vi "Filename Generator.vi"(9 "Measurement Type":string, 10 "Sample Properties:":T1, 11 "Saved Folder:":path=path "C:/1DATA/2011") -> (3 "Filepath Out":path)   [LabVIEW 2012]
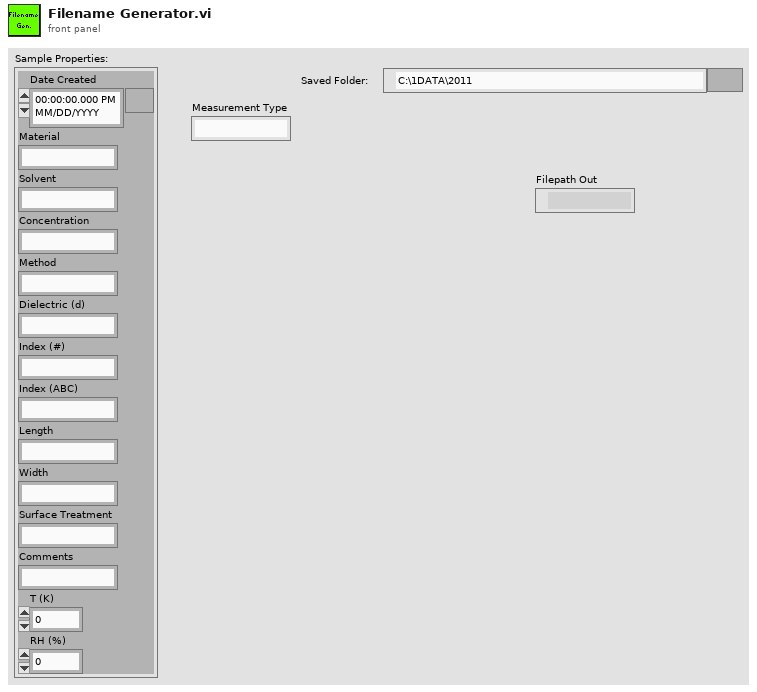
[diagram p1: front panel]
types:
  T1 = cluster{"Date Created":timestamp, "Material":string, "Solvent":string, "Concentration":string, "Method":string, "Dielectric (d)":string, "Index (#)":string, "Index (ABC)":string, "Length":string, "Width":string, "Surface Treatment":string, "Comments":string, "T (K)":dbl, "RH (%)":dbl}
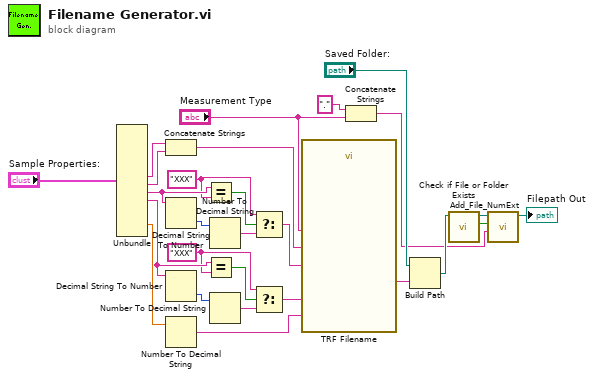
[diagram p0: block diagram]
diagram:
  w22 = "XXX"
  w19 = "XXX"
  n1 = Unbundle("Sample Properties:") -> ("Index (#)"=w14:string, "Index (ABC)"=w15:string, "Length"=w25:string, "Width"=w23:string, "T (K)"=w26:dbl)  [unwired: 9 out]
  n2 = Concatenate Strings(w14, w15) -> (w6:string)
  n3 = Decimal String To Number(string=w25) -> (number=w16:i32)  [unwired: 2 in, 1 out]
  n4 = Decimal String To Number(string=w23) -> (number=w17:i32)  [unwired: 2 in, 1 out]
  n5 = Number To Decimal String(number=w26) -> (decimal integer string=w2:string)  [unwired: 1 in]
  n6 = Equal?(x=w25, y=w19) -> (x = y?=w18:bool)
  n7 = Equal?(x=w23, y=w22) -> (x = y?=w21:bool)
  n8 = Number To Decimal String(number=w16) -> (decimal integer string=w20:string)  [unwired: 1 in]
  n9 = Number To Decimal String(number=w17) -> (decimal integer string=w24:string)  [unwired: 1 in]
  n10 = Select(t=w19, s=w18, f=w20) -> (s? t:f=w4:string)
  n11 = Select(t=w22, s=w21, f=w24) -> (s? t:f=w3:string)
  n12 = call "TRF Filename"("Width"=w3, "Type"="Measurement Type", "Index"=w6, "Length"=w4, "T"=w2) -> ("Result"=w13:string)  [unwired: 9 in, 1 out]
  n13 = Concatenate Strings("." ("string"), "Measurement Type") -> (w7:string)
  n14 = Build Path(base path="Saved Folder:", name or relative path=w13) -> (appended path=w11:path)
  n15 = call <vilib>:"Check if File or Folder Exists.vi"("path"=w11) -> ("file or folder exists?"=w10:bool, "dup path"=w9:path)  [unwired: 8 in, 1 out]
  n16 = call "Add_File_NumExt.vi"("Extension"=w7, "file or folder exists?"=w10, "Path In"=w9) -> ("Path Out"=→"Filepath Out":path)  [unwired: 8 in]
